vi "Create Period Measurement Channel.vi"(6 "index":i32, 7 "measurement edge":T1, 8 "error in (no error)":errorcluster, 9 "default value":bool, 10 "name":string, 11 "Period Measurement Channel in":refnum<class "Period Measurement Channel.lvclass">) -> (0 "error out":errorcluster, 3 "Period Measurement Channel out":refnum<class "Period Measurement Channel.lvclass">)   [LabVIEW 2017, in "Period Measurement Channel.lvclass"]
uses:
  Period Measurement Channel.lvclass
  Measurement Edge.ctl
  Desktop/Scan Engine Sandbox/Channel Classes/Channel/Type.ctl
  Desktop/Scan Engine Sandbox/Channel Classes/Channel/Channel.lvclass
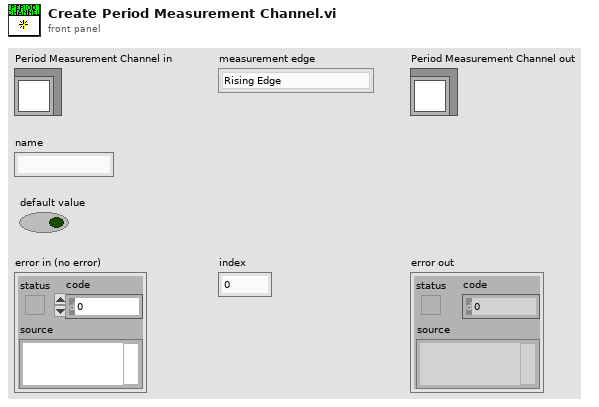
[diagram p1: front panel]
types:
  T1 = typedef "Period Measurement Channel.lvclass/Measurement Edge.ctl" = enum16{"Rising Edge", "Falling Edge"}
  T2 = typedef "Channel.lvclass/Type.ctl" = enum16{"Input", "Output"}
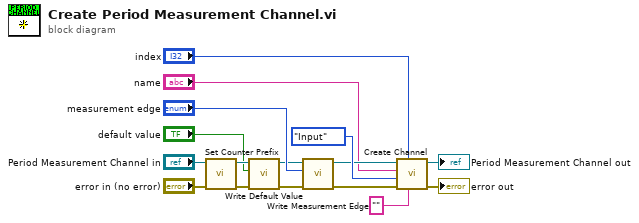
[diagram p0: block diagram]
diagram:
  n1 = call-dynamic "Set Counter Prefix.vi"("error in"="error in (no error)", "counter interface in"="Period Measurement Channel in") -> ("error out"=w3:errorcluster, "counter interface out"=w5:refnum<class "Period Measurement Channel.lvclass">)  [unwired: 8 in]
  n2 = call-dynamic "Write Default Value.vi"("error in"=w3, "default value"="default value", "digital channel in"=w5) -> ("error out"=w2:errorcluster, "digital channel out"=w4:refnum<class "Period Measurement Channel.lvclass">)  [unwired: 7 in]
  n3 = call-dynamic "Write Measurement Edge.vi"("error in"=w2, "measurement edge"="measurement edge", "period measurement channel in"=w4) -> ("error out"=w12:errorcluster, "period measurement channel out"=w11:refnum<class "Period Measurement Channel.lvclass">)  [unwired: 7 in]
  n4 = call-dynamic "Create Channel.vi"("units"="", "index"="index", "error in"=w12, "type"=Type."Input", "name"="name", "channel in"=w11) -> ("error out"=→"error out":errorcluster, "channel out"=→"Period Measurement Channel out":refnum<class "Period Measurement Channel.lvclass">)  [unwired: 4 in]
